vi "Sawtooth Waveform.vi"(5 "offset":dbl format="%.2p", 6 "sampling info":cluster{"Fs":dbl, "#s":dbl}={"Fs"=1000.0, "#s"=1000.0} {"Fs" format="%.2p"}, 7 "reset signal":bool, 8 "error in (no error)":errorcluster, 9 "phase":dbl format="%.2p", 10 "amplitude":dbl=1.0 format="%.2p", 11 "frequency":dbl=10.0 format="%.2p") -> (0 "error out":errorcluster, 3 "signal out":waveform(dbl))   [LabVIEW 2020, in "NI_MABase.lvlib"]
doc: "Generates a waveform containing a sawtooth wave."
uses:
  NI_MABase.lvlib
  NI_AALBase.lvlib
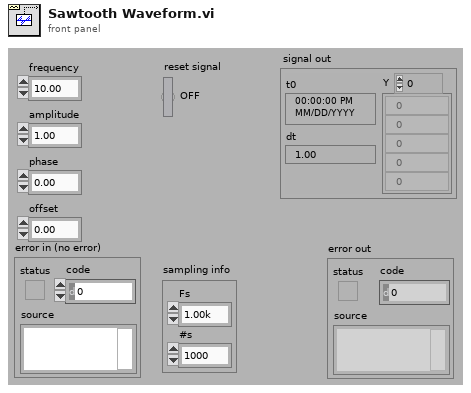
[diagram p1: front panel]
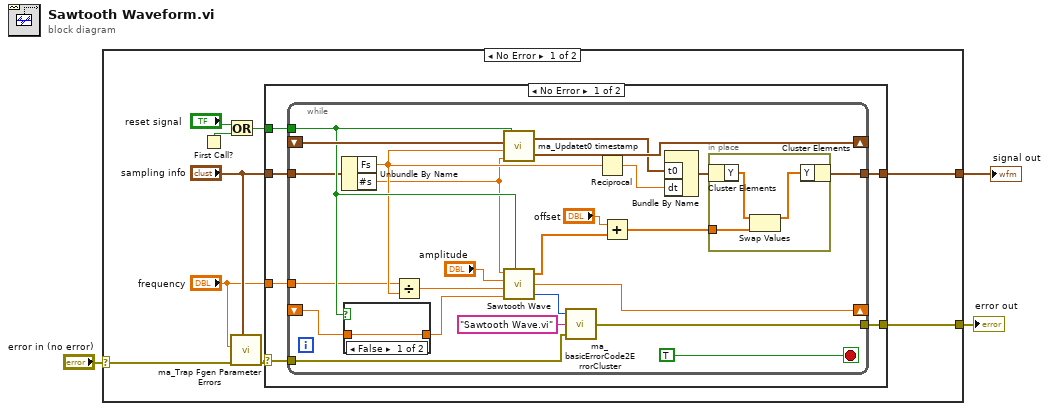
[diagram p0: block diagram]
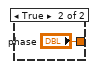
[diagram p2: hidden frame]
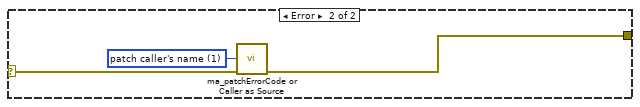
[diagram p3: hidden frame]
diagram:
  n1 = case shown="No Error" "error in (no error)" {
    selector: "error in (no error)" -> [w5 w51]
    tunnel: [w6 w51] -> w3
    tunnel: [w4 _] -> w1
    frame No Error {
      n2 = First Call?() -> (First Call?: T/F=w10:bool)
      n3 = Or(x="reset signal", y=w10) -> (x .or. y?=w11:bool)
      n4 = call "ma_Trap Fgen Parameter Errors.vi"("Sampling info"="sampling info", "error in (no error)"=w5, "frequency"="frequency") -> ("error out"=w9:errorcluster)  [unwired: 8 in]
      n5 = case shown="No Error" w9 {
        selector: w9 -> [w13 w50]
        tunnel: w11 -> [w18 _]
        tunnel: "sampling info" -> [w17 _]
        tunnel: "frequency" -> [w16 _]
        tunnel: [w15 w49] -> w6
        tunnel: [w14 _] -> w4
        frame No Error {
          n6 = while {
            tunnel: w13 -> [w23]
            tunnel: [w20] -> w14
            tunnel: [w24] -> w15
            tunnel: w16 -> [w25]
            tunnel: w17 -> [w26]
            tunnel: w18 -> [w30]
            shift-left: _ -> [w33]
            shift-right: [w35] -> _
            shift-left: _ -> [w39]
            shift-right: [w38] -> _
            stop <- TRUE stop-if-true
            n7 = Unbundle By Name(w26) -> ("Fs"=w28:dbl, "#s"=w27:dbl)
            n8 = case shown="False" w30 {
              tunnel: [w46 "phase"] -> w34
              tunnel: w33 -> [w46 _]
              frame False {
              }
              frame True {
              }
            }
            n9 = Divide(x=w25, y=w28) -> (x/y=w29:dbl)
            n10 = call "ma_Updatet0 timestamp.vi"("samples"=w27, "sampling rate (S/s)"=w28, "tf previous"=w39, "Reset Generation"=w30) -> ("tf new"=w38:timestamp, "t0"=w22:timestamp)
            n11 = call "Sawtooth Wave.vi"("samples"=w27, "amplitude"="amplitude", "frequency"=w29, "phase in"=w34, "reset phase"=w30) -> ("sawtooth wave"=w36:dbl[], "phase out"=w35:dbl, "error"=w42:i32)
            n12 = call "ma_basicErrorCode2ErrorCluster.vi"("error in (no error)"=w23, "subVI name"="Sawtooth Wave.vi" ("subVI Name"), "Error Code"=w42) -> ("error out"=w24:errorcluster)
            n13 = Reciprocal(x=w28) -> (1/x=w32:dbl)
            n14 = Add(x="offset", y=w36) -> (x+y=w19:dbl[])
            n15 = Bundle By Name("t0"=w22, "dt"=w32) -> (w21:waveform(dbl))  [unwired: 1 in]
            n16 = in-place {
              in-place-border: w19 -> [w43]
              n17 = in-place-cluster #1(w21) -> ("Y"=w45:dbl[])
              n18 = Swap Values(12:w45, 14:w43) -> (1:w44:dbl[])  [unwired: 1 in, 1 out]
              n19 = in-place-cluster #1("Y"=w44) -> (w20:waveform(dbl))
            }
          }
        }
        frame Error {
          w48 = u16 1 items=["patch error code", "patch caller's name"] ("operation")
          n20 = call "ma_patchErrorCode or Caller as Source.vi"("error in (no error)"=w50, "operation"=w48) -> ("error out"=w49:errorcluster)  [unwired: 9 in]
        }
      }
    }
    frame Error {
    }
  }
  "error out" <- w3
  "signal out" <- w1
